vi "Job Sequence Executor.vi"(8 "error out":errorcluster, 11 "Test Object":T1={"Program Properties"={"Application Path"=path ""}, "Control Refnum"={"Tree Refnum "=refnum, "Graph1 Refnum"=refnum, "Graph2 Refnum"=refnum, "Temperature Refnum"=refnum, "Sensor Str Refnum"=refnum, "Motor Speed Refnum"=refnum, "Equipment Connected Refnum"=refnum, "Calibrated Refnum"=refnum, "Positioning Refnum"=refnum, "Servo On Refnum"=refnum, "seqPauseButton"=refnum, "seqStartButton"=refnum, "seqStopButton"=refnum}, "Devices"={"Modbus"={"Modbus master instance"=refnum, "Modbus Address"=[{"Session"="Modbus_Write_HR", [{"Key"="Elevator_Position", "value"=310}, {"Key"="Rotation_Speed", "value"=311}, {"Key"="Torque", "value"=312}]}, {"Session"="Modbus_Read_HR", [{"Key"="Elevator_Position", "value"=410}, {"Key"="Rotation_Speed", "value"=411}, {"Key"="Torque", "value"=412}, {"Key"="Temperature", "value"=413}]}, {"Session"="Modbus_Write_Coil", [{"Key"="Servodriver_On", "value"=300}]}, {"Session"="Modbus_Read_Coil", [{"Key"="Servodriver_On", "value"=400}]}]}, "TCP/IP"={"connection ID"=refnum, "Address"=""}, "DAQ Device"={"AI physical channels"="DemoDevice,BID#0/ai0", "AI task out"=0, "AO physical channels"="DemoDevice,BID#0/ai0", "AO task out"=0}}}) -> (0 "error out 2":errorcluster, 3 "Test Object out":T1={"Program Properties"={"Application Path"=path ""}, "Control Refnum"={"Tree Refnum "=refnum, "Graph1 Refnum"=refnum, "Graph2 Refnum"=refnum, "Temperature Refnum"=refnum, "Sensor Str Refnum"=refnum, "Motor Speed Refnum"=refnum, "Equipment Connected Refnum"=refnum, "Calibrated Refnum"=refnum, "Positioning Refnum"=refnum, "Servo On Refnum"=refnum, "seqPauseButton"=refnum, "seqStartButton"=refnum, "seqStopButton"=refnum}, "Devices"={"Modbus"={"Modbus master instance"=refnum, "Modbus Address"=[{"Session"="Modbus_Write_HR", [{"Key"="Elevator_Position", "value"=310}, {"Key"="Rotation_Speed", "value"=311}, {"Key"="Torque", "value"=312}]}, {"Session"="Modbus_Read_HR", [{"Key"="Elevator_Position", "value"=410}, {"Key"="Rotation_Speed", "value"=411}, {"Key"="Torque", "value"=412}, {"Key"="Temperature", "value"=413}]}, {"Session"="Modbus_Write_Coil", [{"Key"="Servodriver_On", "value"=300}]}, {"Session"="Modbus_Read_Coil", [{"Key"="Servodriver_On", "value"=400}]}]}, "TCP/IP"={"connection ID"=refnum, "Address"=""}, "DAQ Device"={"AI physical channels"="DemoDevice,BID#0/ai0", "AI task out"=0, "AO physical channels"="DemoDevice,BID#0/ai0", "AO task out"=0}}})   [LabVIEW 2021]
uses:
  TypeDefs/Tester Object.ctl
  <vilib>/NI/Modbus Library/API/Master/Modbus Master.lvclass
  TypeDefs/UIControlReferences.ctl
  TypeDefs/Devices Cluster.ctl
  Modbus/Modbus Cluster.ctl
  DAQ/DAQNav/DAQNav Cluster.ctl
  FGV Multiplot Action.ctl
  FGV Test Time Action.ctl
  UI Screens/Get Job Attributes Numeric.vi
  UI Screens/Get Job Attributes Boolean.vi
  UI Screens/Get Job Attribute String.vi
  <vilib>/NI/Modbus Library/API/Wrapper/API Main.lvlib
  <vilib>/NI/Modbus Library/API/Wrapper/Create TCP Master.vi
panel:
  out "stop 2":bool
  out "Timer":dbl
  out "Servomotor On/Off":bool
  out "Rotation/Torque":u16
  out "Elevator Positioning":u16
  in  "stop":bool
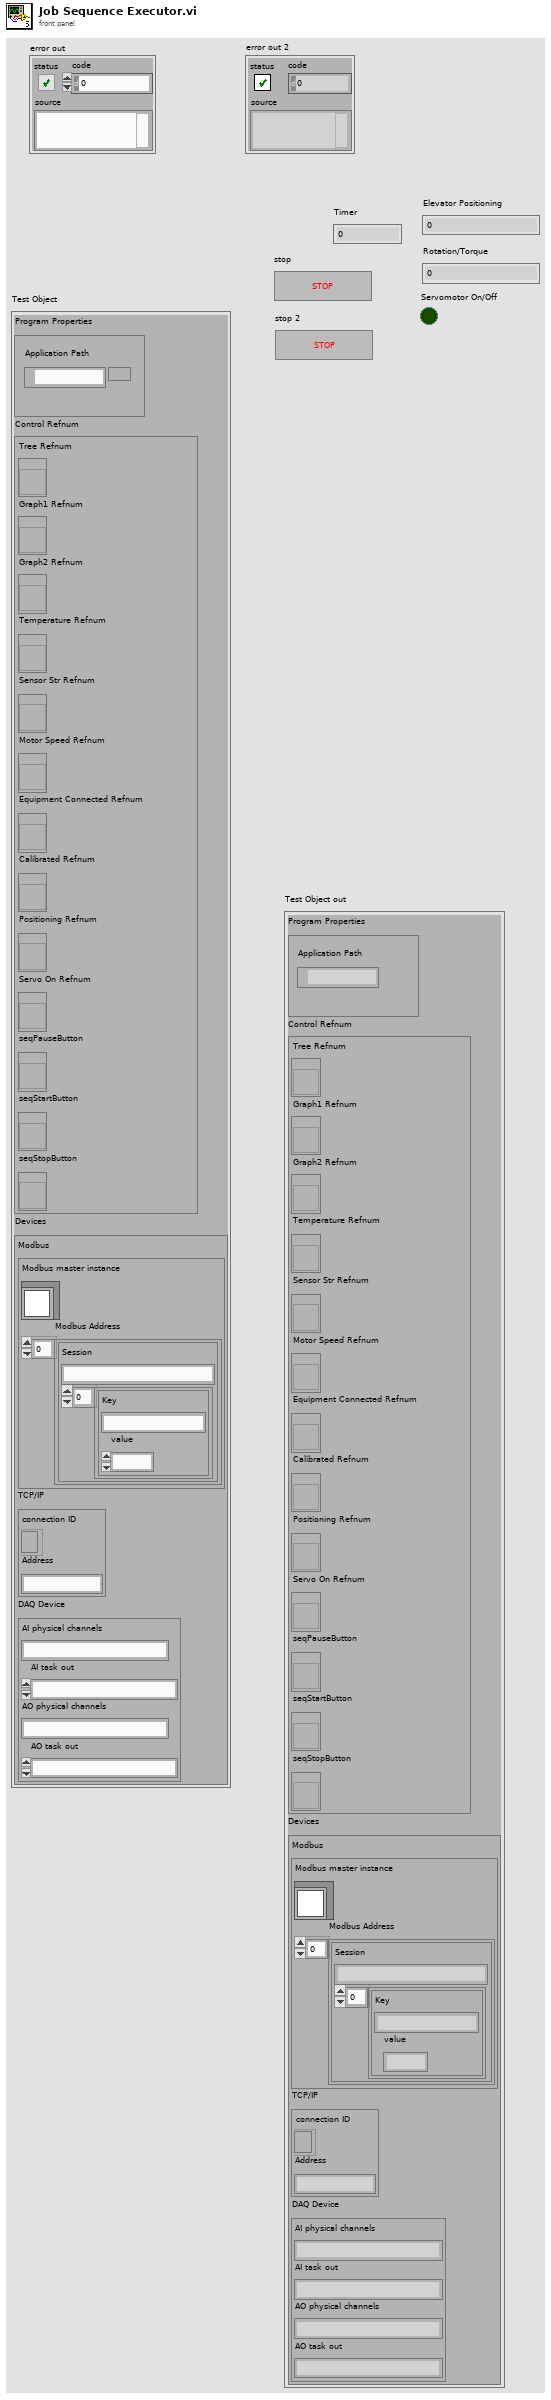
[diagram p1: front panel]
types:
  T1 = typedef "Tester Object.ctl" = cluster{"Program Properties":cluster{"Application Path":path}, "Control Refnum":T2, "Devices":T3}
  T2 = typedef "UIControlReferences.ctl" = cluster{"Tree Refnum ":refnum<vi>, "Graph1 Refnum":refnum<vi>, "Graph2 Refnum":refnum<vi>, "Temperature Refnum":refnum<vi>, "Sensor Str Refnum":refnum<vi>, "Motor Speed Refnum":refnum<vi>, "Equipment Connected Refnum":refnum<vi>, "Calibrated Refnum":refnum<vi>, "Positioning Refnum":refnum<vi>, "Servo On Refnum":refnum<vi>, "seqPauseButton":refnum<vi>, "seqStartButton":refnum<vi>, "seqStopButton":refnum<vi>}
  T3 = typedef "Devices Cluster.ctl" = cluster{"Modbus":T4, "TCP/IP":cluster{"connection ID":refnum<k5>, "Address":string}, "DAQ Device":T5}
  T4 = typedef "Modbus Cluster.ctl" = cluster{"Modbus master instance":refnum<class "Modbus Master.lvclass">, "Modbus Address":cluster{"Session":string, cluster{"Key":string, "value":u32}[]}[]}
  T5 = typedef "DAQNav Cluster.ctl" = cluster{"AI physical channels":string, "AI task out":i32, "AO physical channels":string, "AO task out":i32}
  T6 = cluster{"JOB Item":string, "JOB Attributes":string[][]}[]
  T7 = typedef "FGV Multiplot Action.ctl" = enum16{"Initialize", "Read"}
  T8 = typedef "FGV Test Time Action.ctl" = enum16{"Reset", "Read"}
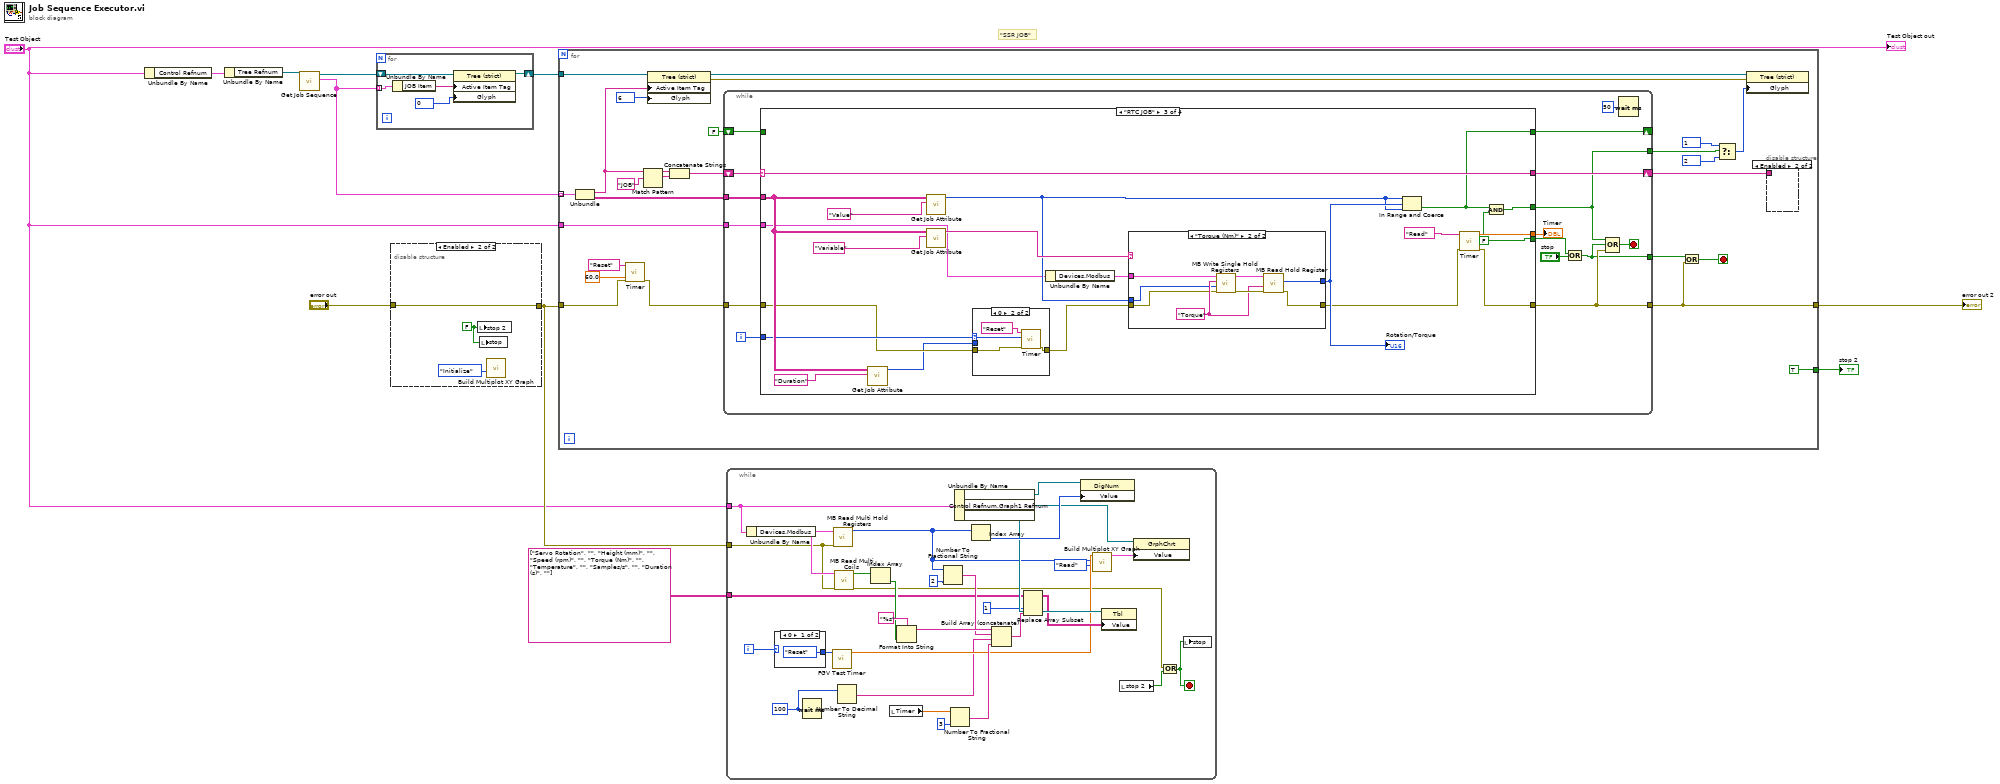
[diagram p0: block diagram]
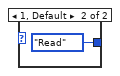
[diagram p2: hidden frame]
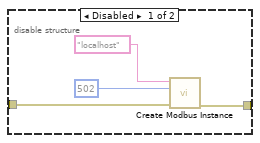
[diagram p3: hidden frame]
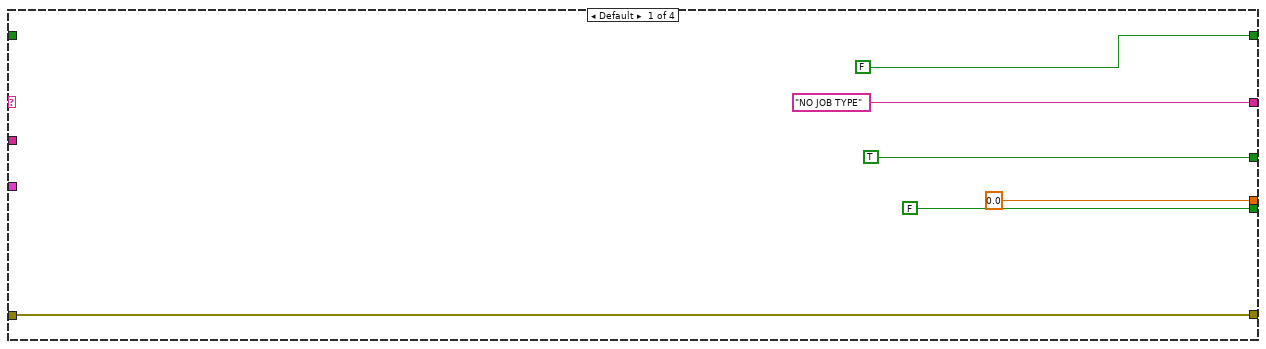
[diagram p4: hidden frame]
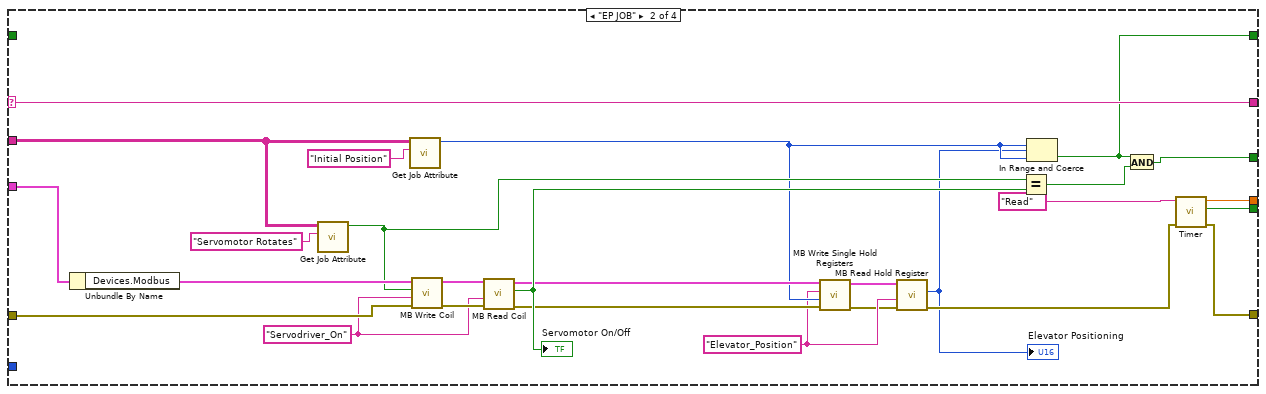
[diagram p5: hidden frame]
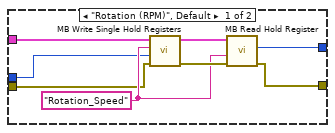
[diagram p7: hidden frame]
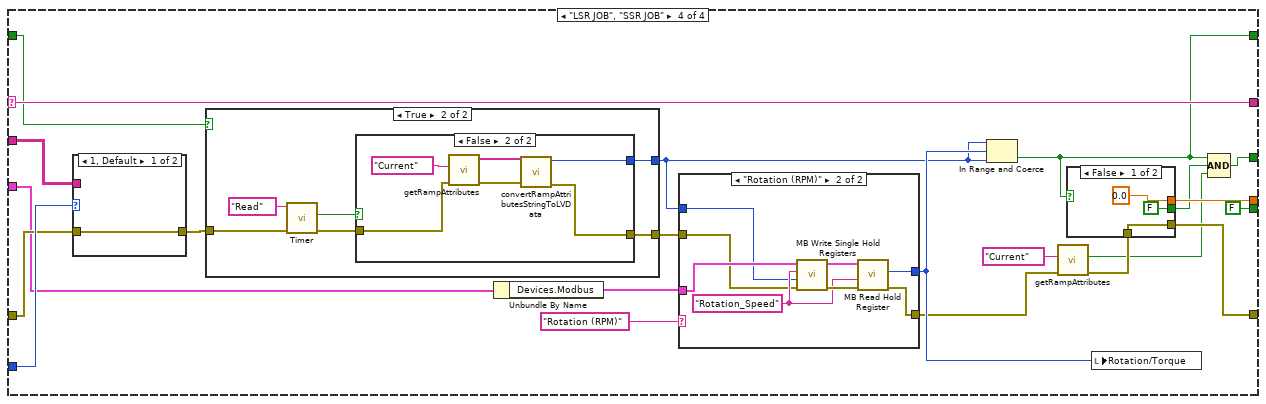
[diagram p8: hidden frame]
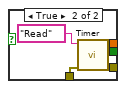
[diagram p9: hidden frame]
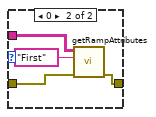
[diagram p10: hidden frame]
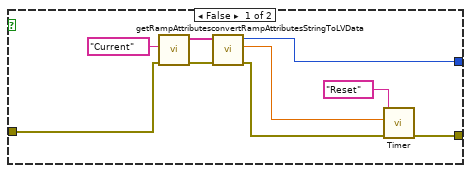
[diagram p11: hidden frame]
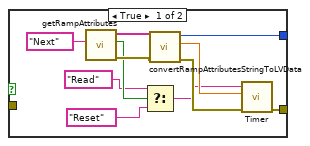
[diagram p12: hidden frame]
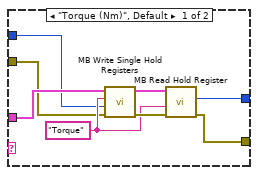
[diagram p13: hidden frame]
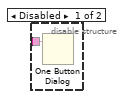
[diagram p14: hidden frame]
diagram:
  # "\"SSR JOB\""
  n1 = Unbundle By Name("Test Object") -> ("Control Refnum"=w2:T2)
  n2 = Unbundle By Name(w2) -> ("Tree Refnum"=w7:refnum<vi>)
  n3 = call "Get Job Sequence.vi"("Job Sequence Tree Reference in"=w7) -> ("JOB  Sequence Array"=w11:T6, "Job Sequence Tree Reference out"=w10:refnum<vi>)  [unwired: 8 in]
  n4 = for {
    tunnel: w11 -> [w16] mode=indexing
    shift-right: [w13] -> w9
    shift-left: w10 -> [w14]
    n5 = Unbundle By Name(w16) -> ("JOB Item"=w15:string)
    n6 = property class="Tree (strict)"(reference=w14, "Active Item Tag"=w15, "Glyph"=0) -> (reference out=w13:refnum<vi>)  [unwired: 1 in, 1 out]
  }
  n7 = disable-structure shown="Enabled" {
    disable-tunnel: "error out" -> [w20 w24]
    disable-tunnel: [w19 w24] -> w5
    frame Disabled {
      n8 = call-poly <vilib>:"Create Modbus Instance.vi"("error in"=w20, "port (502)"=u16 502, "address"="localhost") -> ("error out"=w19:errorcluster, "TCP master instance"=w21:refnum<class "Modbus Master.lvclass">)  [unwired: 7 in]
    }
    frame Enabled {
      w23 = FALSE ("stop 2")
      n9 = local write "stop 2"(w23) -> ()
      n10 = local write "stop"(w23) -> ()
      n11 = call "Build Multiplot XY Graph.vi"("FGV Build Multiplot XY"=FGV_Multiplot_Action."Initialize") -> ()  [unwired: 9 in, 2 out]
    }
  }
  n12 = for {
    tunnel: w11 -> [w50] mode=indexing
    tunnel: w9 -> [w42]
    tunnel: [w33] -> w6
    tunnel: w5 -> [w30]
    tunnel: [TRUE] -> w3
    tunnel: "Test Object" -> [w25]
    stop <- w32 stop-if-true
    n13 = Unbundle(w50) -> ("JOB Item"=w41:string, "JOB Attributes"=w48:string[][])
    n14 = call "Timer.vi"("error in (no error)"=w30, "Time Target (s)"=60.0, "Timer Action"="Reset") -> ("error out"=w29:errorcluster)  [unwired: 6 in, 2 out]
    n15 = Match Pattern(string=w41, regular expression="JOB") -> (before substring=w45:string, match substring=w46:string)  [unwired: 1 in, 2 out]
    n16 = property class="Tree (strict)"(reference=w42, "Active Item Tag"=w41, "Glyph"=6) -> (reference out=w40:refnum<vi>, error out=w35:errorcluster)  [unwired: 1 in]
    n17 = Concatenate Strings(w45, w46) -> (w44:string)
    n18 = while {
      tunnel: w48 -> [w66]
      tunnel: [w54] -> w36
      shift-right: [w65] -> w47
      shift-left: w44 -> [w64]
      tunnel: [w61] -> w33
      tunnel: w29 -> [w62]
      tunnel: [w57] -> w34
      shift-right: [w53] -> _
      shift-left: FALSE -> [w52]
      tunnel: w25 -> [w51]
      i -> [w63]
      stop <- w60 stop-if-true
      n19 = case shown="\"RTC JOB\"" w64 {
        selector: w64 -> [_ w99 w121 w164]
        tunnel: w66 -> [_ w98 w113 w149]
        tunnel: ["NO JOB TYPE" w99 w121 w164] -> w65
        tunnel: [FALSE w88 w102 w145] -> w53
        tunnel: w63 -> [_ _ w111 w152]
        tunnel: [w69 w93 w116 w163] -> w61
        tunnel: w62 -> [w69 w97 w110 w151]
        tunnel: [TRUE w90 w105 w154] -> w54
        tunnel: [FALSE ("Time has Elapsed") w92 FALSE ("Time has Elapsed") FALSE ("Time has Elapsed")] -> w58
        tunnel: [0.0 ("Present (s)") w89 w106 w161] -> w56
        tunnel: w52 -> [_ _ _ w148]
        tunnel: w51 -> [_ w87 w101 w144]
        frame Default {
        }
        frame "EP JOB" {
          w77 = "Elevator_Position" ("Control Variable")
          w82 = "Servodriver_On" ("Key")
          n20 = Unbundle By Name(w87) -> ("Devices.Modbus"=w86:T4)
          n21 = call-poly "Get Job Attribute.vi"("element"="Servomotor Rotates", "JOB Attributes"=w98) -> ("Cell Value"=w85:bool)  [unwired: 9 in]
          n22 = call-poly "Get Job Attribute.vi"("Attribute"="Initial Position" ("element"), "JOB Attributes"=w98) -> ("Cell String"=w78:u16)  [unwired: 9 in]
          n23 = call "MB Write Coil.vi"("error in (no error)"=w97, "Key"=w82, "Write Value"=w85, "Devices"=w86) -> ("error out"=w83:errorcluster, "Devices Out"=w84:T4)  [unwired: 6 in]
          n24 = call "MB Read Coil.vi"("error in (no error)"=w83, "Key"=w82, "Devices"=w84) -> ("error out"=w79:errorcluster, "coils"=w81:bool, "Devices out"=w80:T4)  [unwired: 6 in]
          "Servomotor On/Off" <- w81
          n25 = call "MB Write Single Hold Registers.vi"("error in (no error)"=w79, "Write Hold Register"=w78, "Control Variable"=w77, "Devices"=w80) -> ("error out"=w76:errorcluster, "Devices out"=w75:T4)  [unwired: 6 in]
          n26 = call "MB Read Hold Register.vi"("error in"=w76, "Key"=w77, "Devices"=w75) -> ("error out"=w74:errorcluster, "Register value"=w73:u16)  [unwired: 6 in, 1 out]
          "Elevator Positioning" <- w73
          n27 = Equal?(x=w85, y=w81) -> (x = y?=w91:bool)
          n28 = In Range and Coerce(upper limit=w78, x=w73, lower limit=w78) -> (In Range?=w88:bool)  [unwired: 1 out]
          n29 = And(x=w88, y=w91) -> (x .and. y?=w90:bool)
          n30 = call "Timer.vi"("error in (no error)"=w74, "Timer Action"="Read") -> ("error out"=w93:errorcluster, "Time has Elapsed"=w92:bool, "Present (s)"=w89:dbl)  [unwired: 7 in]
        }
        frame "RTC JOB" {
          n31 = call-poly "Get Job Attribute.vi"("Attribute"="Duration" ("element"), "JOB Attributes"=w113) -> ("Cell String"=w109:u16)  [unwired: 9 in]
          n32 = call-poly "Get Job Attribute.vi"("Attribute"="Value" ("element"), "JOB Attributes"=w113) -> ("Cell String"=w107:u16)  [unwired: 9 in]
          n33 = call-poly "Get Job Attribute.vi"("element"="Variable", "JOB Attributes"=w113) -> ("Cell String"=w112:string)  [unwired: 9 in]
          n34 = case shown="0" w111 {
            tunnel: w110 -> [w122 w125]
            tunnel: w109 -> [_ w124]
            tunnel: [w122 w123] -> w108
            frame Default {
            }
            frame 0 {
              n35 = call "Timer.vi"("error in (no error)"=w125, "Time Target (s)"=w124, "Timer Action"="Reset") -> ("error out"=w123:errorcluster)  [unwired: 6 in, 2 out]
            }
          }
          n36 = Unbundle By Name(w101) -> ("Devices.Modbus"=w100:T4)
          n37 = case shown="\"Torque (Nm)\"" w112 {
            tunnel: w100 -> [w131 w139]
            tunnel: w108 -> [w127 w136]
            tunnel: [w129 w138] -> w120
            tunnel: [w130 w137] -> w117
            tunnel: w107 -> [w128 w135]
            frame "Rotation (RPM)", Default {
              w132 = "Rotation_Speed" ("Control Variable")
              n38 = call "MB Write Single Hold Registers.vi"("error in (no error)"=w127, "Write Hold Register"=w128, "Control Variable"=w132, "Devices"=w131) -> ("error out"=w134:errorcluster, "Devices out"=w133:T4)  [unwired: 6 in]
              n39 = call "MB Read Hold Register.vi"("error in"=w134, "Key"=w132, "Devices"=w133) -> ("error out"=w130:errorcluster, "Register value"=w129:u16)  [unwired: 6 in, 1 out]
            }
            frame "Torque (Nm)" {
              w140 = "Torque" ("Control Variable")
              n40 = call "MB Write Single Hold Registers.vi"("error in (no error)"=w136, "Write Hold Register"=w135, "Control Variable"=w140, "Devices"=w139) -> ("error out"=w142:errorcluster, "Devices out"=w141:T4)  [unwired: 6 in]
              n41 = call "MB Read Hold Register.vi"("error in"=w142, "Key"=w140, "Devices"=w141) -> ("error out"=w137:errorcluster, "Register value"=w138:u16)  [unwired: 6 in, 1 out]
            }
          }
          "Rotation/Torque" <- w120
          n42 = In Range and Coerce(upper limit=w107, x=w120, lower limit=w107) -> (In Range?=w102:bool)  [unwired: 1 out]
          n43 = call "Timer.vi"("error in (no error)"=w117, "Timer Action"="Read") -> ("error out"=w116:errorcluster, "Time has Elapsed"=w104:bool, "Present (s)"=w106:dbl)  [unwired: 7 in]
          n44 = And(x=w102, y=w104) -> (x .and. y?=w105:bool)
        }
        frame "LSR JOB", "SSR JOB" {
          n45 = case shown="1, Default" w152 {
            tunnel: w151 -> [w173 w176]
            tunnel: [w173 w175] -> w150
            tunnel: w149 -> [_ w174]
            frame 1, Default {
            }
            frame 0 {
              n46 = call "getRampAttributes.vi"("error in (no error)"=w176, "FGV Count Action"="First", "LSR JOB Attribute"=w174) -> ("error out"=w175:errorcluster)  [unwired: 6 in, 2 out]
            }
          }
          n47 = case shown="True" w148 {
            tunnel: [w184 w190] -> w158
            tunnel: [w183 w192] -> w159
            tunnel: w150 -> [w179 w189]
            frame False {
              n48 = call "getRampAttributes.vi"("error in (no error)"=w179, "FGV Count Action"="Current") -> ("error out"=w181:errorcluster, "subarray"=w185:string[])  [unwired: 7 in, 1 out]
              n49 = call "convertRampAttributesStringToLVData.vi"("error in (no error)"=w181, "Job Ramp Array"=w185) -> ("error out"=w180:errorcluster, "Duration"=w182:dbl, "Setpoint"=w184:u16)  [unwired: 7 in]
              n50 = call "Timer.vi"("error in (no error)"=w180, "Time Target (s)"=w182, "Timer Action"="Reset") -> ("error out"=w183:errorcluster)  [unwired: 6 in, 2 out]
            }
            frame True {
              n51 = call "Timer.vi"("error in (no error)"=w189, "Timer Action"="Read") -> ("error out"=w188:errorcluster, "Time has Elapsed"=w187:bool)  [unwired: 7 in, 1 out]
              n52 = case shown="False" w187 {
                tunnel: [w202 w207] -> w192
                tunnel: [w197 w206] -> w190
                tunnel: w188 -> [_ w204]
                frame True {
                  n53 = call "getRampAttributes.vi"("FGV Count Action"="Next") -> ("error out"=w200:errorcluster, "Last?"=w196:bool, "subarray"=w201:string[])  [unwired: 8 in]
                  n54 = Select(t="Read" ("Timer Action"), s=w196, f="Reset" ("Timer Action")) -> (s? t:f=w193:string)
                  n55 = call "convertRampAttributesStringToLVData.vi"("error in (no error)"=w200, "Job Ramp Array"=w201) -> ("error out"=w199:errorcluster, "Duration"=w198:dbl, "Setpoint"=w197:u16)  [unwired: 7 in]
                  n56 = call "Timer.vi"("error in (no error)"=w199, "Time Target (s)"=w198, "Timer Action"=w193) -> ("error out"=w202:errorcluster)  [unwired: 6 in, 2 out]
                }
                frame False {
                  n57 = call "getRampAttributes.vi"("error in (no error)"=w204, "FGV Count Action"="Current") -> ("error out"=w208:errorcluster, "subarray"=w209:string[])  [unwired: 7 in, 1 out]
                  n58 = call "convertRampAttributesStringToLVData.vi"("error in (no error)"=w208, "Job Ramp Array"=w209) -> ("error out"=w207:errorcluster, "Setpoint"=w206:u16)  [unwired: 7 in, 1 out]
                }
              }
            }
          }
          n59 = Unbundle By Name(w144) -> ("Devices.Modbus"=w143:T4)
          n60 = case shown="\"Rotation (RPM)\"" "Rotation (RPM)" ("Cell String") {
            tunnel: w143 -> [w214 w222]
            tunnel: [w210 w218] -> w162
            tunnel: [w213 w221] -> w156
            tunnel: w158 -> [w211 w219]
            tunnel: w159 -> [w212 w220]
            frame "Torque (Nm)", Default {
              w215 = "Torque" ("Control Variable")
              n61 = call "MB Write Single Hold Registers.vi"("error in (no error)"=w212, "Write Hold Register"=w211, "Control Variable"=w215, "Devices"=w214) -> ("error out"=w217:errorcluster, "Devices out"=w216:T4)  [unwired: 6 in]
              n62 = call "MB Read Hold Register.vi"("error in"=w217, "Key"=w215, "Devices"=w216) -> ("error out"=w213:errorcluster, "Register value"=w210:u16)  [unwired: 6 in, 1 out]
            }
            frame "Rotation (RPM)" {
              w223 = "Rotation_Speed" ("Control Variable")
              n63 = call "MB Write Single Hold Registers.vi"("error in (no error)"=w220, "Write Hold Register"=w219, "Control Variable"=w223, "Devices"=w222) -> ("error out"=w225:errorcluster, "Devices out"=w224:T4)  [unwired: 6 in]
              n64 = call "MB Read Hold Register.vi"("error in"=w225, "Key"=w223, "Devices"=w224) -> ("error out"=w221:errorcluster, "Register value"=w218:u16)  [unwired: 6 in, 1 out]
            }
          }
          n65 = In Range and Coerce(upper limit=w158, x=w162, lower limit=w158) -> (In Range?=w145:bool)  [unwired: 1 out]
          n66 = call "getRampAttributes.vi"("error in (no error)"=w156, "FGV Count Action"="Current") -> ("error out"=w153:errorcluster, "Last?"=w146:bool)  [unwired: 7 in, 1 out]
          n67 = case shown="False" w145 {
            tunnel: [w165 w172] -> w163
            tunnel: [0.0 ("Present (s)") w171] -> w161
            tunnel: [FALSE ("Time has Elapsed") w170] -> w155
            tunnel: w153 -> [w165 w169]
            frame False {
            }
            frame True {
              n68 = call "Timer.vi"("error in (no error)"=w169, "Timer Action"="Read") -> ("error out"=w172:errorcluster, "Time has Elapsed"=w170:bool, "Present (s)"=w171:dbl)  [unwired: 7 in]
            }
          }
          n69 = local write "Rotation/Torque"(w162) -> ()
          n70 = Compound Arithmetic op=AND(w145, w155, w146) -> (w154:bool)
        }
      }
      "Timer" <- w56
      n71 = Or(x=w58, y="stop") -> (x .or. y?=w57:bool)
      n72 = Compound Arithmetic op=OR(w54, w57, w61) -> (w60:bool)
      n73 = Wait (ms)(milliseconds to wait=u32 50) -> ()  [unwired: 1 out]
    }
    n74 = Or(x=w34, y=w33) -> (x .or. y?=w32:bool)
    n75 = Select(t=1, s=w36, f=2) -> (s? t:f=w37:i32)
    n76 = property class="Tree (strict)"(reference=w40, error in=w35, "Glyph"=w37) -> ()  [unwired: 2 out]
    n77 = disable-structure shown="Enabled" {
      disable-tunnel: w47 -> [w226 _]
      frame Disabled {
        n78 = One Button Dialog(message=w226) -> ()  [unwired: 1 in, 1 out]
      }
      frame Enabled {
      }
    }
  }
  "error out 2" <- w6
  "stop 2" <- w3
  n79 = while {
    tunnel: w5 -> [w231]
    tunnel: string[][] [["Servo Rotation", ""], ["Height (mm)", ""], ["Speed (rpm)", ""], ["Torque (Nm)", ""], ["Temperature", ""], ["Samples/s", ""], ["Duration (s)", ""]] ("Sensors") -> [w247]
    tunnel: "Test Object" -> [w229]
    i -> [w237]
    stop <- w239 stop-if-true
    w228 = u32 100 ("milliseconds to wait")
    n80 = Unbundle By Name(w229) -> ("Devices.Modbus"=w232:T4)
    n81 = case shown="0" w237 {
      tunnel: [FGV_Test_Time_Action."Reset" ("FGV Test Time") FGV_Test_Time_Action."Read" ("FGV Test Time")] -> w236
      frame 0 {
      }
      frame 1, Default {
      }
    }
    n82 = Wait (ms)(milliseconds to wait=w228) -> ()  [unwired: 1 out]
    n83 = call "FGV Test Timer.vi"("FGV Test Time"=w236) -> ("Time (s)"=w235:dbl)  [unwired: 10 in]
    n84 = call "MB Read Multi Hold Registers.vi"("error in"=w231, "Modbus"=w232) -> ("Register Values"=w233:u16[])  [unwired: 8 in, 1 out]
    n85 = call "MB Read Multi Coils.vi"("error in (no error)"=w231, "Devices"=w232) -> ("error out"=w230:errorcluster, "coils"=w252:bool[])  [unwired: 7 in, 1 out]
    n86 = Number To Decimal String(number=w228) -> (decimal integer string=w227:string)  [unwired: 1 in]
    n87 = Index Array(array=w252) -> (element=w251:bool)  [unwired: 1 in]
    n88 = local read "Timer"() -> (w243:dbl)
    n89 = Format Into String(format string="%s", w251) -> (resulting string=w249:string)  [unwired: 2 in, 1 out]
    n90 = Number To Fractional String(number=w233, precision (6)=i16 2) -> (F-format string=w248:string[])  [unwired: 2 in]
    n91 = Number To Fractional String(number=w243, precision (6)=i16 3) -> (F-format string=w241:string)  [unwired: 2 in]
    n92 = Unbundle By Name(w229) -> ("Control Refnum.Positioning Refnum"=w257:refnum<vi>, "Control Refnum.Graph1 Refnum"=w255:refnum<vi>, "Control Refnum.Sensor Str Refnum"=w254:refnum<vi>)
    n93 = Index Array(array=w233) -> (element=w256:u16)  [unwired: 1 in]
    n94 = Build Array (concatenate)(w249, w248, w227, w241) -> (w246:string[])
    n95 = Replace Array Subset(array=w247, new element=w246, index (col)=1 ("disabled index (col)")) -> (w244:string[][])  [unwired: 1 in]
    n96 = property class="DigNum"(reference=w257, "Value"=w256) -> ()  [unwired: 1 in, 2 out]
    n97 = call "Build Multiplot XY Graph.vi"("FGV Build Multiplot XY"=FGV_Multiplot_Action."Read", "Sensor Array in"=w233, "Time"=w235) -> ("Multiplot XY Array"=w238:cluster{dbl[], dbl[]}[])  [unwired: 7 in, 1 out]
    n98 = property class="Tbl"(reference=w254, "Value"=w244) -> ()  [unwired: 1 in, 2 out]
    n99 = local read "stop 2"() -> (w240:bool)
    n100 = property class="GrphChrt"(reference=w255, "Value"=w238) -> ()  [unwired: 1 in, 2 out]
    n101 = Or(x=w230, y=w240) -> (x .or. y?=w239:bool)
    n102 = local write "stop"(w239) -> ()
  }
  "Test Object out" <- "Test Object"
